vi "Generate Chip Select.vi"(10 "Address":u16 format="%04x", 11 "Memory Map in":refnum<class "Memory Map.lvclass">) -> (1 "VIA /CS":bool, 2 "EEPROM /CS":bool, 3 "RAM /CS":bool)   [LabVIEW 2021, in "Memory Map.lvclass"]
uses:
  Memory Map.lvclass
  Memory Map.lvclass/Memory Map.ctl
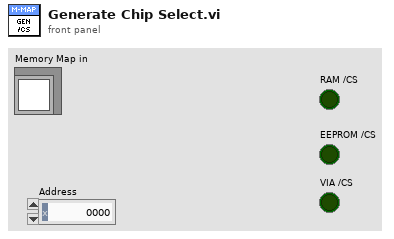
[diagram p1: front panel]
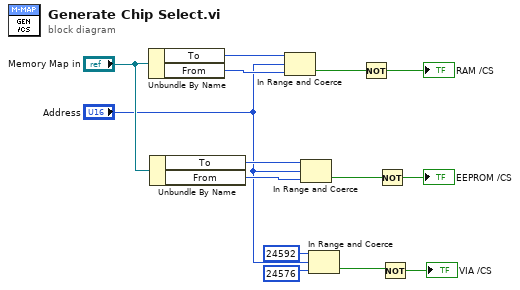
[diagram p0: block diagram]
diagram:
  n1 = Unbundle By Name("Memory Map in") -> ("To"=w13:u16, "From"=w12:u16)
  n2 = Unbundle By Name("Memory Map in") -> ("To"=w8:u16, "From"=w7:u16)
  n3 = In Range and Coerce(upper limit=w13, x="Address", lower limit=w12) -> (In Range?=w11:bool)  [unwired: 1 out]
  n4 = In Range and Coerce(upper limit=w8, x="Address", lower limit=w7) -> (In Range?=w9:bool)  [unwired: 1 out]
  n5 = In Range and Coerce(upper limit=u16 24592, x="Address", lower limit=u16 24576 ("upper limit")) -> (In Range?=w2:bool)  [unwired: 1 out]
  n6 = Not(x=w11) -> (.not. x?=→"RAM /CS":bool)
  n7 = Not(x=w9) -> (.not. x?=→"EEPROM /CS":bool)
  n8 = Not(x=w2) -> (.not. x?=→"VIA /CS":bool)
